vi "Export Drivetrain Acquired Data.vi"(10 "string":string, 11 "Array":dbl[][](array[numeric])) -> ()   [LabVIEW 2015]
uses:
  <vilib>/Utility/file.llb/Write Delimited Spreadsheet (DBL).vi
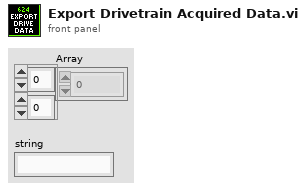
[diagram p1: front panel]
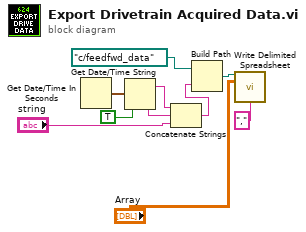
[diagram p0: block diagram]
diagram:
  n1 = Get Date/Time In Seconds() -> (seconds since 1Jan1904=w3:timestamp)
  n2 = Get Date/Time String(seconds (now)=w3, want seconds? (F)=TRUE) -> (date string=w5:string, time string=w6:string)  [unwired: 1 in]
  n3 = Concatenate Strings(w5, w6, "string") -> (w7:string)
  n4 = Build Path(base path=path "c/feedfwd_data", name or relative path=w7) -> (appended path=w1:path)
  n5 = call-poly <vilib>:"Write Delimited Spreadsheet.vi"("file path (dialog if empty)"=w1, "2D data"="Array", "delimiter (\\t)"="," ("delimiter (\\t)")) -> ()  [unwired: 11 in, 2 out]
